vi "Teleop.vi"(10 "Match Info":T1={"Autonomous Elapsed Seconds"=0.0, "TeleOp Elapsed Seconds"=0.0, "Disabled Elapsed Seconds"=0.0, "Visited Autonomous"=FALSE, "Visited TeleOp"=FALSE, "Visited Disabled"=FALSE, "Autonomous Settings"={"Autonomous Style"=enum."Independent", "VI Refnum"=refnum}}, 11 "Call Context":T2) -> ()   [LabVIEW 2019]
doc: "This VI is called for each TeleOp packet received from the DS where the robot is not disabled. It is often used to read from the joysticks and update I/O or to update setpoints for timed control loops. It should complete and return within 20 milliseconds or it may miss DS packets."
uses:
  <vilib>/Rock Robotics/WPI/DriverStation/WPI_DriverStationDerivedRobotMode.ctl
  <vilib>/Rock Robotics/WPI/DriverStation/WPI_DriverStationMatch Info.ctl
  <vilib>/Rock Robotics/WPI/Utilities/WPI_GetSetVariantRefNum.vi
panel:
  out "Angle":u16
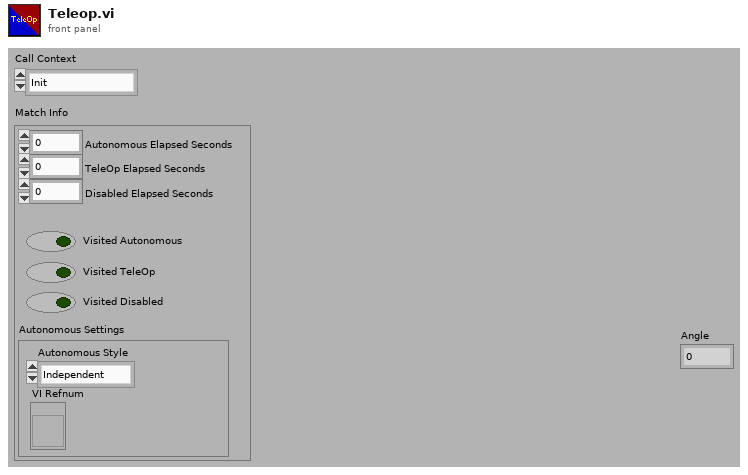
[diagram p1: front panel]
types:
  T1 = typedef "WPI_DriverStationMatch Info.ctl" = cluster{"Autonomous Elapsed Seconds":dbl, "TeleOp Elapsed Seconds":dbl, "Disabled Elapsed Seconds":dbl, "Visited Autonomous":bool, "Visited TeleOp":bool, "Visited Disabled":bool, "Autonomous Settings":cluster{"Autonomous Style":enum16{"Iterative", "Independent"}, "VI Refnum":refnum<vi>}}
  T2 = typedef "WPI_DriverStationDerivedRobotMode.ctl" = enum16{"Init", "Execute", "Stop"}
  T3 = typedef "WPI_JoystickDevRef.ctl" = cluster{"Device":T4}
  T4 = typedef "WPI_JoystickDeviceEnum.ctl" = enum16{"USB 0", "USB 1", "USB 2", "USB 3", "USB 4", "USB 5"}
  T5 = typedef "WPI_RobotDriveDevRef.ctl" = cluster{"DevStatus":errorcluster, "Motors[]":T6[], "Square Inputs":bool, "Max Output":dbl}
  T6 = typedef "WPI_MotorControlDeviceRef.ctl" = cluster{"DeviceStatus":errorcluster, "Type":T7, "PWM":cluster{"PWM Channel":T8, "DeadBand":T9}, "CAN":cluster{"Device Number":u8, "SetOutput VI Ref":variant, "GetOutput VI Ref":variant, "Enable VI Ref":variant, "Disable VI Ref":variant, "Data":variant}, "Invert":bool, "DIO PWM":cluster{"PWM \"Enable\" Channel":T8, "DIOChannel":T10, "PWM Rate":dbl}}
  T7 = typedef "WPI_MotorControlType.ctl" = enum16{"PWM", "CAN", "DIO PWM"}
  T8 = typedef "FPGA_DIOPWMChannel.ctl" = enum8{"PWM 0", "PWM 1", "PWM 2", "PWM 3", "PWM 4", "PWM 5", "PWM 6", "PWM 7", "PWM 8", "PWM 9", "PWM MXP 0", "PWM MXP 1", "PWM MXP 2", "PWM MXP 3", "PWM MXP 4", "PWM MXP 5", "PWM MXP 6", "PWM MXP 7", "PWM MXP 8", "PWM MXP 9", "Invalid"}
  T9 = typedef "WPI_PWMDeadband.ctl" = cluster{"Name":string, "maxPositivePwm":i32, "minPositivePwm":i32, "centerPwm":i32, "maxNegativePwm":i32, "minNegativePwm":i32, "angularRange":u16}
  T10 = typedef "FPGA_DIOChannel.ctl" = enum8{"DIO 0", "DIO 1", "DIO 2", "DIO 3", "DIO 4", "DIO 5", "DIO 6", "DIO 7", "DIO 8", "DIO 9", "DIO MXP 0", "DIO MXP 1", "DIO MXP 2", "DIO MXP 3", "DIO MXP 4", "DIO MXP 5", "DIO MXP 6", "DIO MXP 7", "DIO MXP 8", "DIO MXP 9", "DIO MXP 10", "DIO MXP 11", "DIO MXP 12", "DIO MXP 13", "DIO MXP 14", "DIO MXP 15", "SPI Port CS1", "SPI Port CS2", "SPI Port CS3", "SPI Port MISO", "SPI Port MOSI", "Invalid"}
  T11 = cluster{"JoystickDevRef":T3, "RobotDriveDevRef":T5}
  T12 = typedef "WPI_ServoDeviceRef.ctl" = cluster{"DeviceStatus":errorcluster, "PWM Channel":T8, "DeadBand":T9}
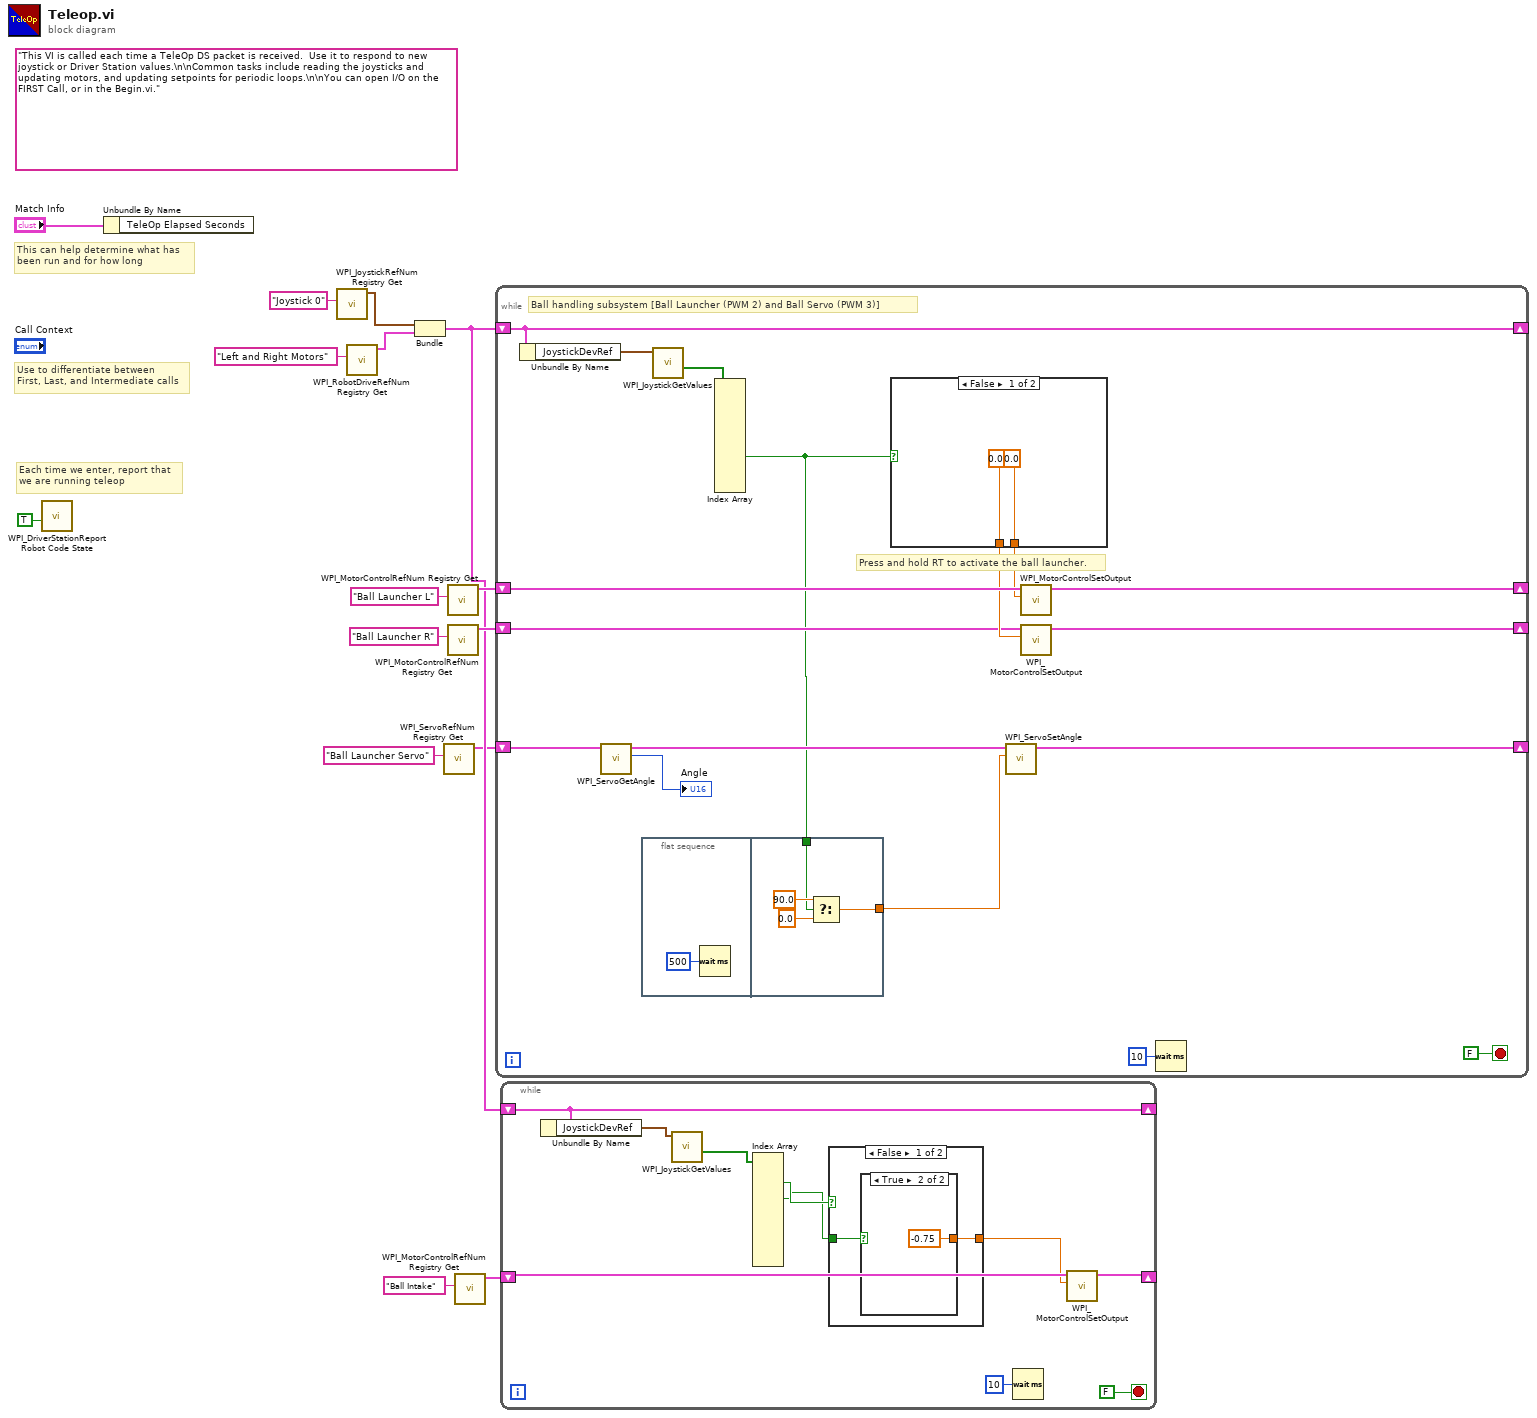
[diagram p0: block diagram]
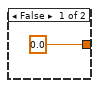
[diagram p2: hidden frame]
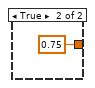
[diagram p3: hidden frame]
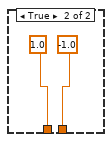
[diagram p4: hidden frame]
diagram:
  (unwired) "This VI is called each time a TeleOp DS packet is received.  Use it to respond to new joystick or Driver Station values.\n\nCommon tasks include reading the joysticks and updating motors, and updating setpoints for periodic loops.\n\nYou can open I/O on the FIRST Call, or in the Begin.vi."
  # "Each time we enter, report that\nwe are running teleop"
  # "Use to differentiate between\nFirst, Last, and Intermediate calls"
  # "This can help determine what has\nbeen run and for how long"
  n1 = call <vilib>:"WPI_DriverStationReport Robot Code State.vi"("TeleOp"=TRUE ("Autonomous")) -> ()  [unwired: 10 in, 1 out]
  n2 = Unbundle By Name("Match Info") -> ()  [unwired: 1 out]
  n3 = call <vilib>:"WPI_JoystickRefNum Registry Get.vi"("refnum name"="Joystick 0") -> ("JoystickDevRef"=w10:T3)  [unwired: 9 in, 1 out]
  n4 = call <vilib>:"WPI_RobotDriveRefNum Registry Get.vi"("refnum name"="Left and Right Motors") -> ("RobotDriveDevRef"=w11:T5)  [unwired: 9 in, 1 out]
  n5 = Bundle("JoystickDevRef"=w10, "RobotDriveDevRef"=w11) -> (w3:T11)  [unwired: 1 in]
  n6 = call <vilib>:"WPI_ServoRefNum Registry Get.vi"("refnum name"="Ball Launcher Servo") -> ("ServoDeviceRef"=w1:T12)  [unwired: 9 in, 1 out]
  n7 = call <vilib>:"WPI_MotorControlRefNum Registry Get.vi"("refnum name"="Ball Launcher L") -> ("MotorControlDevRef"=w9:T6)  [unwired: 9 in, 1 out]
  n8 = call <vilib>:"WPI_MotorControlRefNum Registry Get.vi"("refnum name"="Ball Launcher R") -> ("MotorControlDevRef"=w6:T6)  [unwired: 9 in, 1 out]
  n9 = call <vilib>:"WPI_MotorControlRefNum Registry Get.vi"("refnum name"="Ball Intake") -> ("MotorControlDevRef"=w4:T6)  [unwired: 9 in, 1 out]
  n10 = while {
    shift-right: [w31] -> _
    shift-left: w3 -> [w31]
    shift-right: [w23] -> _
    shift-left: w9 -> [w28]
    shift-right: [w22] -> _
    shift-left: w6 -> [w24]
    shift-right: [w18] -> _
    shift-left: w1 -> [w21]
    stop <- FALSE stop-if-true
    # "Ball handling subsystem [Ball Launcher (PWM 2) and Ball Servo (PWM 3)]"
    # "Press and hold RT to activate the ball launcher."
    n11 = Unbundle By Name(w31) -> ("JoystickDevRef"=w30:T3)
    n12 = call <vilib>:"WPI_ServoGetAngle.vi"("ServoDeviceRef"=w21) -> ("ServoDeviceRef"=w19:T12, "Angle"=→"Angle":u16)  [unwired: 7 in, 1 out]
    n13 = flat-sequence {
      tunnel: w17 -> [w35]
      tunnel: [w34] -> w16
      frame #0 {
        n14 = Wait (ms)(milliseconds to wait=u32 500) -> ()  [unwired: 1 out]
      }
      frame #1 {
        n15 = Select(t=90.0, s=w35, f=0.0) -> (s? t:f=w34:dbl)
      }
    }
    n16 = call <vilib>:"WPI_JoystickGetValues.vi"("JoystickDevRef"=w30) -> ("Buttons"=w29:bool[])  [unwired: 6 in, 4 out]
    n17 = Index Array(array=w29) -> (element #8=w17:bool)  [unwired: 12 in, 11 out]
    n18 = case shown="False" w17 {
      tunnel: [0.0 ("Output") -1.0 ("Output")] -> w27
      tunnel: [0.0 ("Output") 1.0 ("Output")] -> w25
      frame False {
      }
      frame True {
      }
    }
    n19 = call <vilib>:"WPI_ServoSetAngle.vi"("Angle"=w16, "ServoDeviceRef"=w19) -> ("ServoDeviceRef"=w18:T12)  [unwired: 8 in, 1 out]
    n20 = call <vilib>:"WPI_MotorControlSetOutput.vi"("Output"=w27, "MotorControlDevRef"=w28) -> ("MotorControlDevRef"=w23:T6)  [unwired: 7 in, 2 out]
    n21 = call <vilib>:"WPI_MotorControlSetOutput.vi"("Output"=w25, "MotorControlDevRef"=w24) -> ("MotorControlDevRef"=w22:T6)  [unwired: 7 in, 2 out]
    n22 = Wait (ms)(milliseconds to wait=u32 10) -> ()  [unwired: 1 out]
  }
  n23 = while {
    shift-right: [w47] -> _
    shift-left: w4 -> [w46]
    shift-right: [w51] -> _
    shift-left: w3 -> [w51]
    stop <- FALSE stop-if-true
    n24 = Unbundle By Name(w51) -> ("JoystickDevRef"=w50:T3)
    n25 = call <vilib>:"WPI_JoystickGetValues.vi"("JoystickDevRef"=w50) -> ("Buttons"=w49:bool[])  [unwired: 6 in, 4 out]
    n26 = Index Array(array=w49) -> (element #2=w48:bool, element #4=w44:bool)  [unwired: 12 in, 10 out]
    n27 = case shown="False" w48 {
      tunnel: [w53 0.75 ("Output")] -> w45
      tunnel: w44 -> [w52 _]
      frame False {
        n28 = case shown="True" w52 {
          tunnel: [0.0 ("Output") -0.75 ("Output")] -> w53
          frame False {
          }
          frame True {
          }
        }
      }
      frame True {
      }
    }
    n29 = Wait (ms)(milliseconds to wait=u32 10) -> ()  [unwired: 1 out]
    n30 = call <vilib>:"WPI_MotorControlSetOutput.vi"("Output"=w45, "MotorControlDevRef"=w46) -> ("MotorControlDevRef"=w47:T6)  [unwired: 7 in, 2 out]
  }
